vi "CMD_Lift.vi"(1 "Line":string) -> (0 "Done":bool)   [LabVIEW 2017, in "Apple script.lvlib"]
uses:
  Apple script.lvlib
  Robot Global Data.vi
panel:
  in  "Parameters":i32[](array[numeric])=[1, 2]
  in  "Subcommands":string[](array[string])=["to", "to"]
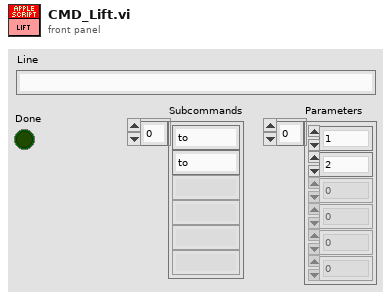
[diagram p1: front panel]
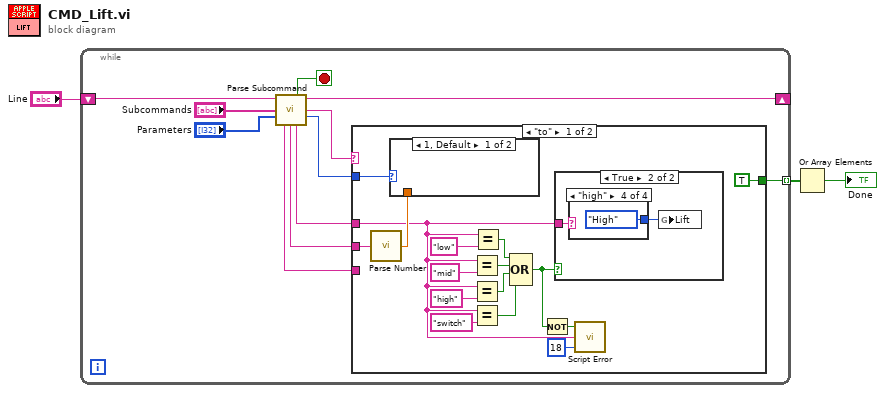
[diagram p0: block diagram]
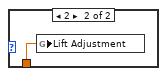
[diagram p2: hidden frame]
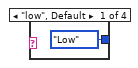
[diagram p4: hidden frame]
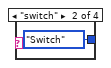
[diagram p5: hidden frame]
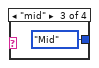
[diagram p6: hidden frame]
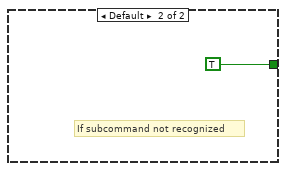
[diagram p7: hidden frame]
diagram:
  n1 = while {
    shift-right: [w11] -> _
    shift-left: "Line" -> [w14]
    tunnel: [w4] -> w2 mode=indexing
    stop <- w10 stop-if-true
    n2 = call "Parse Subcommand.vi"("Text In"=w14, "Subcommands"="Subcommands", "Parameters"="Parameters") -> ("Done"=w10:bool, "Text Out"=w11:string, "Subcommand"=w9:string, "# of Parameters"=w8:i32, "Parameter 3"=w5:string, "Parameter 2"=w6:string, "Parameter 1"=w7:string)  [unwired: 6 in]
    n3 = case shown="\"to\"" w9 {
      tunnel: w8 -> [w21 _]
      tunnel: w7 -> [w15 _]
      tunnel: w6 -> [w20 _]
      tunnel: w5 -> [_ _]
      tunnel: [TRUE TRUE] -> w4
      frame "to" {
        n4 = call "Parse Number.vi"("String"=w20) -> ("Number"=w19:dbl)
        n5 = case shown="1, Default" w21 {
          tunnel: w19 -> [_ w31]
          frame 1, Default {
          }
          frame 2 {
            n6 = global write "Robot Global Data.vi" "Lift Adjustment"(w31) -> ()
          }
        }
        n7 = Equal?(x=w15, y="mid") -> (x = y?=w25:bool)
        n8 = Equal?(x=w15, y="high") -> (x = y?=w24:bool)
        n9 = Equal?(x=w15, y="switch") -> (x = y?=w16:bool)
        n10 = Equal?(x=w15, y="low") -> (x = y?=w26:bool)
        n11 = Compound Arithmetic op=OR(w26, w25, w24, w16) -> (w23:bool)
        n12 = Not(x=w23) -> (.not. x?=w18:bool)
        n13 = case shown="True" w23 {
          tunnel: w15 -> [_ w33]
          frame False {
          }
          frame True {
            n14 = case shown="\"high\"" w33 {
              tunnel: [enum16{"Low", "Switch", "Mid", "High"}."Low" ("Lift") enum16{"Low", "Switch", "Mid", "High"}."Switch" ("Lift") enum16{"Low", "Switch", "Mid", "High"}."Mid" ("Lift") enum16{"Low", "Switch", "Mid", "High"}."High" ("Lift")] -> w32
              frame "low", Default {
              }
              frame "switch" {
              }
              frame "mid" {
              }
              frame "high" {
              }
            }
            n15 = global write "Robot Global Data.vi" "Lift"(w32) -> ()
          }
        }
        n16 = call "Script Error.vi"("Error?"=w18, "Error Details"=w15, "Error Code"=18) -> ()  [unwired: 2 in, 1 out]
      }
      frame Default {
        # "If subcommand not recognized"
      }
    }
  }
  n17 = Or Array Elements(Boolean array=w2) -> (logical OR=→"Done":bool)
